vi "SVPO AC & DC Level.vi"   [LabVIEW 2017, in "SoundVib_VibrationLevel.lvlib"]
doc: "Computes the AC level and DC level of a signal. Wire data to the <B>scaled signal [EU]</B> input to determine the polymorphic instance to use or manually select the instance."
uses:
  <vilib>/addons/Sound and Vibration/svt_Level/SoundVib_VibrationLevel.lvlib
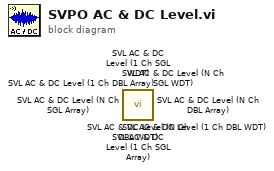
[diagram p0: block diagram]
diagram:
  n1 = call <vilib>:"SVL AC & DC Level (N Ch DBL WDT).vi"() -> ()  [unwired: 9 in, 3 out]
  n2 = call <vilib>:"SVL AC & DC Level (N Ch SGL WDT).vi"() -> ()  [unwired: 9 in, 3 out]
  n3 = call <vilib>:"SVL AC & DC Level (N Ch SGL Array).vi"() -> ()  [unwired: 9 in, 3 out]
  n4 = call <vilib>:"SVL AC & DC Level (N Ch DBL Array).vi"() -> ()  [unwired: 9 in, 3 out]
  n5 = call <vilib>:"SVL AC & DC Level (1 Ch DBL Array).vi"() -> ()  [unwired: 9 in, 3 out]
  n6 = call <vilib>:"SVL AC & DC Level (1 Ch SGL WDT).vi"() -> ()  [unwired: 9 in, 3 out]
  n7 = call <vilib>:"SVL AC & DC Level (1 Ch SGL Array).vi"() -> ()  [unwired: 9 in, 3 out]
  n8 = call <vilib>:"SVL AC & DC Level (1 Ch DBL WDT).vi"() -> ()  [unwired: 9 in, 3 out]
